vi "Get_VI_Refnum.vi"(0 "Application_Directory":path, 2 "Type_Specifier_VI_Refnum":refnum<vi>, 5 "VI_Name":path=path "SubVIs/Password_Popup.vi", 11 "Error_In":errorcluster) -> (4 "VI_Out":refnum<vi>, 15 "Error_Out":errorcluster)   [LabVIEW 2023]
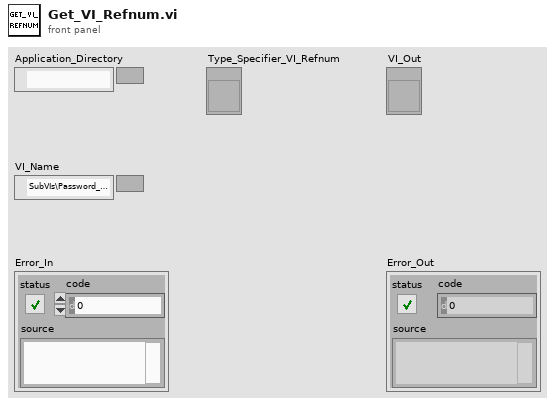
[diagram p1: front panel]
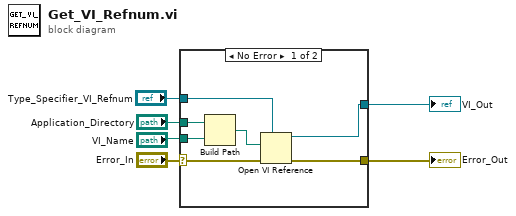
[diagram p0: block diagram]
diagram:
  n1 = case shown="No Error" "Error_In" {
    selector: "Error_In" -> [w8 w15]
    tunnel: "Application_Directory" -> [w13 _]
    tunnel: [w11 w15] -> w5
    tunnel: "Type_Specifier_VI_Refnum" -> [w10 w14]
    tunnel: [w9 w14] -> w3
    tunnel: "VI_Name" -> [w7 _]
    frame No Error {
      n2 = Build Path(base path=w13, name or relative path=w7) -> (appended path=w12:path)
      n3 = Open VI Reference(type specifier VI Refnum (for type only)=w10, vi path=w12, error in (no error)=w8) -> (vi reference=w9:refnum<vi>, error out=w11:errorcluster)  [unwired: 3 in]
    }
    frame Error {
    }
  }
  "Error_Out" <- w5
  "VI_Out" <- w3
